vi "SubPanelBasicFlow.vi"(11 "error in (no error)":errorcluster) -> (15 "error out":errorcluster)   [LabVIEW 2016, in "DronaTest.lvlib"]
uses:
  DronaTest.lvlib
  APIs/Stimulus/ControlValue/ValueSignalByPathString.vi
  APIs/Assert/AssertControlValue/Equal.vi
  <vilib>/addons/_JKI Toolkits/Caraya/classes/Test/Test.lvclass
  Drona.lvlib
  APIs/Stimulus/ControlValue/ControlValue.lvlib
  APIs/Assert/AssertControlValue/AssertControlValue.lvlib
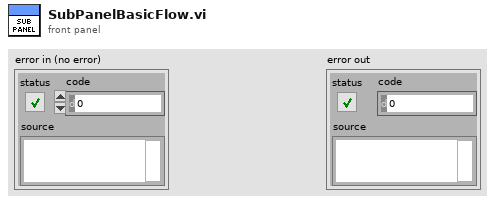
[diagram p1: front panel]
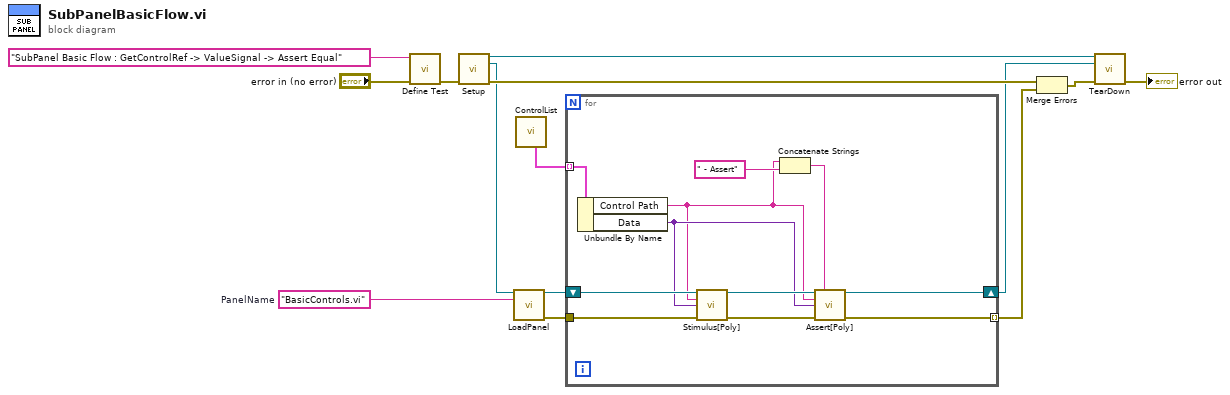
[diagram p0: block diagram]
diagram:
  w8 = "BasicControls.vi"  # PanelName
  n1 = call <vilib>:"Define Test.vi"("error in (no error)"="error in (no error)", "Label (VI Title)"="SubPanel Basic Flow : GetControlRef -> ValueSignal -> Assert Equal") -> ("error out"=w11:errorcluster)  [unwired: 9 in]
  n2 = call "Setup.vi"("error in (no error)"=w11) -> ("Application Ref"=w3:refnum<vi>, "VI out"=w2:refnum<vi>, "error out"=w5:errorcluster)  [unwired: 12 in]
  n3 = call "LoadPanel.vi"("VI in"=w2, "Panel Name"=w8) -> ("VI out"=w7:refnum<vi>, "error out"=w6:errorcluster)  [unwired: 12 in]
  n4 = call "ControlList.vi"() -> ("SubPanel"=w9:cluster{"Control Path":string, "Data":variant}[])  [unwired: 6 in, 5 out]
  n5 = for {
    shift-right: [w25] -> w1
    shift-left: w7 -> [w21]
    tunnel: [w16] -> w14 mode=indexing
    tunnel: w9 -> [w22] mode=indexing
    tunnel: w6 -> [w15]
    n6 = Unbundle By Name(w22) -> ("Control Path"=w17:string, "Data"=w20:variant)
    n7 = call-poly "Stimulus[Poly].vi"("VI Reference In"=w21, "Control Path"=w17, "Value (Signaling)"=w20, "error in"=w15) -> ("VI Reference Out"=w23:refnum<vi>, "error out"=w24:errorcluster)  [unwired: 10 in]
    n8 = Concatenate Strings(w17, " - Assert" ("string")) -> (w18:string)
    n9 = call-poly "Assert[Poly].vi"("VI Reference In"=w23, "Test Label"=w18, "Control Path"=w17, "Control Value"=w20, "Error In"=w24) -> ("VI Reference Out"=w25:refnum<vi>, "Error Out"=w16:errorcluster)  [unwired: 9 in]
  }
  n10 = Merge Errors(w5, w14) -> (w12:errorcluster)
  n11 = call "TearDown.vi"("Application Ref"=w3, "VI in"=w1, "error in (no error)"=w12) -> ("error out"=→"error out":errorcluster)  [unwired: 12 in]
